vi "FourFlippingCoins.vi"() -> ()   [LabVIEW 2015]
uses:
  <vilib>/Analysis/NI_AALBase.lvlib
panel:
  out "Histogram Y":T1(graph)
  in  "Number of Trials":dbl
  out "Number of Heads":dbl
  out "Coin 4":bool
  out "Coin 3":bool
  out "Coin 2":bool
  out "Coin 1":bool
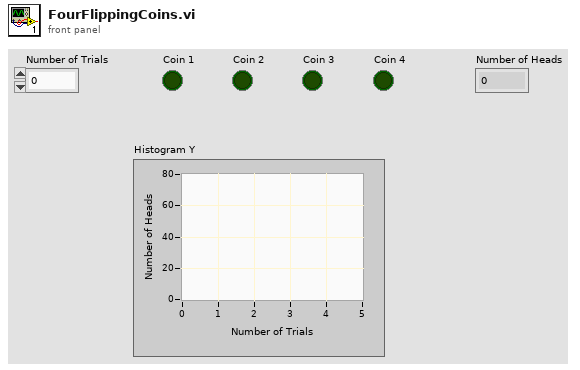
[diagram p1: front panel]
types:
  T1 = cluster{"X Values":dbl[], "Histogram: h(x)":i32[]}
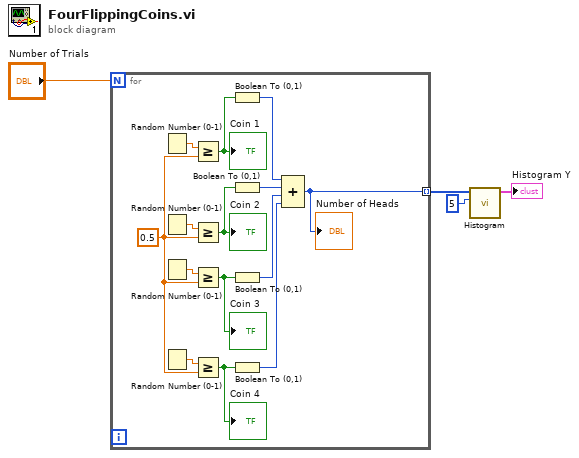
[diagram p0: block diagram]
diagram:
  n1 = for {
    N: "Number of Trials" -> [_]
    tunnel: [w5] -> w3 mode=indexing
    w17 = 0.5
    n2 = Random Number (0-1)() -> (number: 0 to 1=w16:dbl)
    n3 = Random Number (0-1)() -> (number: 0 to 1=w15:dbl)
    n4 = Random Number (0-1)() -> (number: 0 to 1=w14:dbl)
    n5 = Random Number (0-1)() -> (number: 0 to 1=w13:dbl)
    n6 = Greater Or Equal?(x=w16, y=w17) -> (x >= y?=w12:bool)
    "Coin 1" <- w12
    n7 = Greater Or Equal?(x=w15, y=w17) -> (x >= y?=w11:bool)
    "Coin 2" <- w11
    n8 = Greater Or Equal?(x=w14, y=w17) -> (x >= y?=w10:bool)
    "Coin 3" <- w10
    n9 = Greater Or Equal?(x=w13, y=w17) -> (x >= y?=w9:bool)
    "Coin 4" <- w9
    n10 = Boolean To (0,1)(Boolean=w12) -> (0, 1=w18:i16)
    n11 = Boolean To (0,1)(Boolean=w11) -> (0, 1=w8:i16)
    n12 = Boolean To (0,1)(Boolean=w10) -> (0, 1=w7:i16)
    n13 = Boolean To (0,1)(Boolean=w9) -> (0, 1=w6:i16)
    n14 = Compound Arithmetic op=ADD(w18, w8, w7, w6) -> (w5:i16)
    "Number of Heads" <- w5
  }
  n15 = call <vilib>:"Histogram.vi"("intervals"=5, "X"=w3) -> ("Histogram Graph"=→"Histogram Y":T1)  [unwired: 6 in, 3 out]
